vi "DrawCrosshair.vi"(8 "Y":dbl, 9 "X":dbl, 11 "new picture in":picture) -> (1 "Center":cluster{dbl, dbl}, 3 "new picture out":picture)   [LabVIEW 2021]
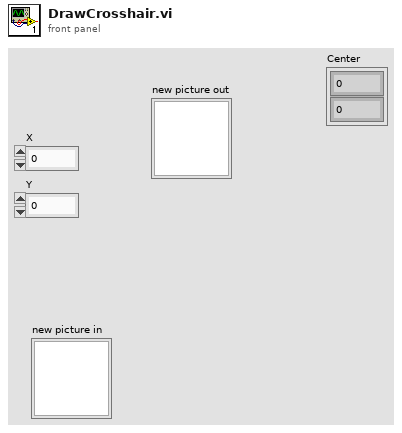
[diagram p1: front panel]
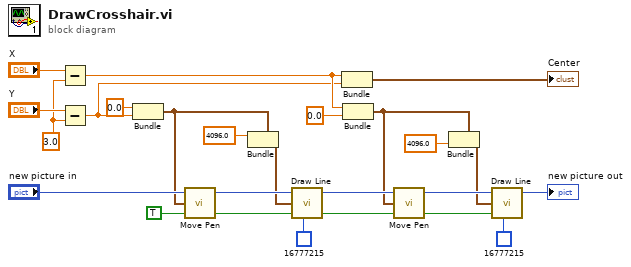
[diagram p0: block diagram]
diagram:
  w4 = 3.0
  w7 = TRUE ("absolute coordinates?(T)")
  n1 = Subtract(x="X", y=w4) -> (x-y=w3:dbl)
  n2 = Subtract(x="Y", y=w4) -> (x-y=w2:dbl)
  n3 = Bundle(0.0, w2) -> (w17:cluster{dbl, dbl})  [unwired: 1 in]
  n4 = call <vilib>:"Move Pen.vi"("absolute coordinates?(T)"=w7, "new position"=w17, "picture"="new picture in") -> ("new picture"=w20:picture)  [unwired: 2 in]
  n5 = Bundle(cluster=w17, 4096.0) -> (w16:cluster{dbl, dbl})  [unwired: 1 in]
  n6 = call <vilib>:"Draw Line.vi"("picture"=w20, "end point"=w16, "absolute coordinates?(T)"=w7, "color(black)"=u32 16777215) -> ("new picture"=w14:picture)  [unwired: 5 in]
  n7 = Bundle(w3, w2) -> (→"Center":cluster{dbl, dbl})  [unwired: 1 in]
  n8 = Bundle(w3, 0.0) -> (w10:cluster{dbl, dbl})  [unwired: 1 in]
  n9 = call <vilib>:"Move Pen.vi"("absolute coordinates?(T)"=w7, "new position"=w10, "picture"=w14) -> ("new picture"=w12:picture)  [unwired: 2 in]
  n10 = Bundle(cluster=w10, 4096.0) -> (w8:cluster{dbl, dbl})  [unwired: 1 in]
  n11 = call <vilib>:"Draw Line.vi"("picture"=w12, "end point"=w8, "absolute coordinates?(T)"=w7, "color(black)"=u32 16777215) -> ("new picture"=→"new picture out":picture)  [unwired: 5 in]
